vi "Init-FileHandler.vi"(5 "Formatter.lvclass":refnum<class "Formatter.lvclass">, 6 "Flush Timeout (5 s)":dbl=5.0, 7 "Filepath":path, 8 "error in":errorcluster, 9 "Level":T1, 10 "Name":string, 11 "FileHandler":refnum<class "FileHandler.lvclass">) -> (0 "error out":errorcluster, 3 "FileHandler out":refnum<class "FileHandler.lvclass">)   [LabVIEW 2016, in "hse-logger.lvlib" / "FileHandler.lvclass"]
doc: "Initiates a new FileHandler-object with a name, log-level and a filepath for the log-file.\nThe handler processes LogRecords only if the level of the handler is greater or equal to the level of the LogRecord.\n\n____\n(c) HAMPEL SOFTWARE ENGINEERING"
uses:
  FileHandler.lvclass
  LogLevel.ctl
  Formatter/Formatter.lvclass
  FileHandler.lvclass/FileHandler.ctl
  hse-logger.lvlib
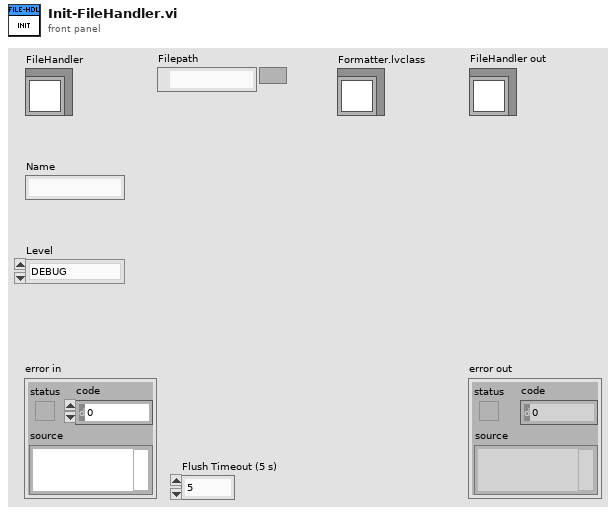
[diagram p1: front panel]
types:
  T1 = typedef "hse-logger.lvlib/LogLevel.ctl" = enum16{"DEBUG", "INFO", "WARNING", "ERROR", "CRITICAL"}
  T2 = enum16{"open", "replace", "create", "open or create", "replace or create", "replace or create with confirmation"}
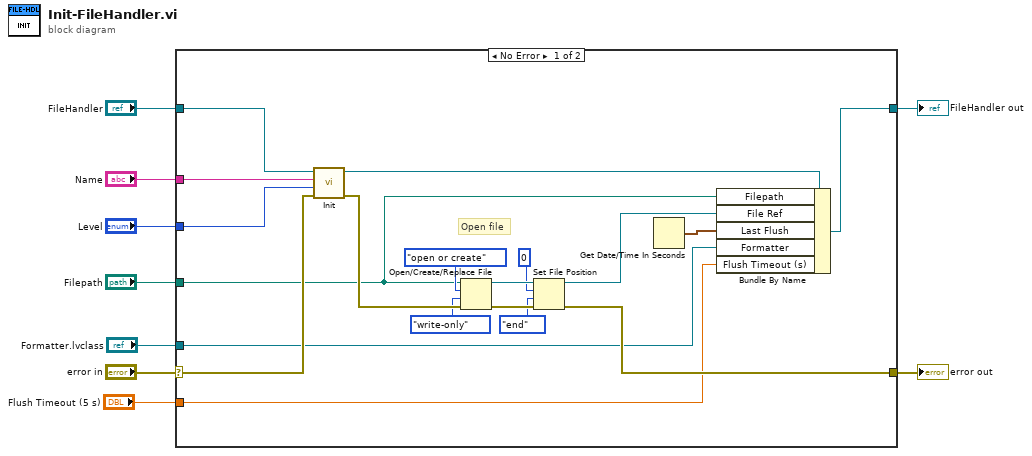
[diagram p0: block diagram]
diagram:
  n1 = case shown="No Error" "error in" {
    selector: "error in" -> [w27 w30]
    tunnel: [w18 w30] -> w8
    tunnel: [w26 w29] -> w7
    tunnel: "Name" -> [w17 _]
    tunnel: "Level" -> [w16 _]
    tunnel: "Filepath" -> [w19 _]
    tunnel: "FileHandler" -> [w15 w29]
    tunnel: "Flush Timeout (5 s)" -> [w11 _]
    tunnel: "Formatter.lvclass" -> [w10 _]
    frame No Error {
      # "Open file"
      n2 = call-dynamic "Init.vi"("error in"=w27, "Level"=w16, "Name"=w17, "Handler"=w15) -> ("error out"=w28:errorcluster, "Handler out"=w14:refnum<class "FileHandler.lvclass">)  [unwired: 6 in]
      n3 = Open/Create/Replace File(file path (use dialog)=w19, error in=w28, operation (0:open)=T2."open or create", access (0:read/write)=enum16{"read/write", "read-only", "write-only"}."write-only") -> (refnum out=w23:refnum<file>, error out=w24:errorcluster)  [unwired: 2 in, 1 out]
      n4 = Set File Position(offset (in bytes) (0)=i64 0, refnum=w23, from (0:start)=enum16{"start", "end", "current"}."end", error in=w24) -> (refnum out=w13:refnum<file>, error out=w18:errorcluster)
      n5 = Get Date/Time In Seconds() -> (seconds since 1Jan1904=w12:timestamp)
      n6 = Bundle By Name(cluster=w14, "Filepath"=w19, "File Ref"=w13, "Last Flush"=w12, "Formatter"=w10, "Flush Timeout (s)"=w11) -> (w26:refnum<class "FileHandler.lvclass">)
    }
    frame Error {
    }
  }
  "error out" <- w8
  "FileHandler out" <- w7
